vi "AMI1700eth_get.vi"(7 "command":string="MEAS:HE:CONT\n", 8 "error in":errorcluster, 11 "conn_id_in":refnum<k5>) -> (0 "error out":errorcluster, 3 "conn_id_out":refnum<k5>, 4 "status":bool, 5 "string":string)   [LabVIEW 2019]
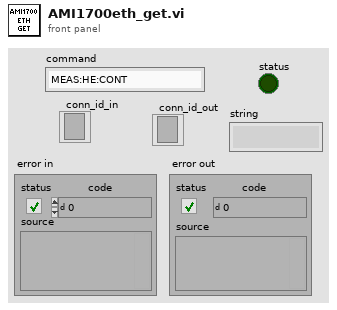
[diagram p1: front panel]
types:
  T1 = enum16{"Standard", "Buffered", "CRLF", "Immediate"}
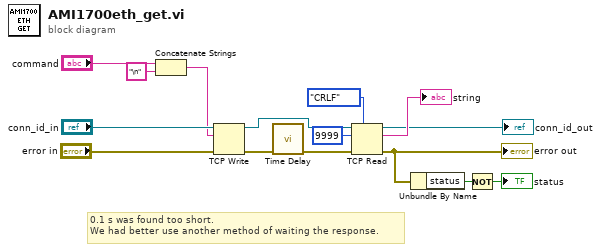
[diagram p0: block diagram]
diagram:
  # "0.1 s was found too short.\nWe had better use another method of waiting the response."
  n1 = Concatenate Strings("command", "\n" ("string")) -> (w6:string)
  n2 = TCP Write(connection ID="conn_id_in", data in=w6, error in (no error)="error in") -> (connection ID out=w12:refnum<k5>, error out=w14:errorcluster)  [unwired: 1 in, 1 out]
  n3 = call "Time Delay"("error in (no error)"=w14) -> ("error out"=w13:errorcluster)  [unwired: 10 in]
  n4 = TCP Read(connection ID=w12, bytes to read=9999, error in (no error)=w13, 7:T1."CRLF" ("mode (standard)")) -> (connection ID out=→"conn_id_out":refnum<k5>, data out=→"string":string, error out=w3:errorcluster)  [unwired: 1 in]
  "error out" <- w3
  n5 = Unbundle By Name(w3) -> ("status"=w2:bool)
  n6 = Not(x=w2) -> (.not. x?=→"status":bool)
